vi "Increment Stage.vi"(11 "Circle the Wagons in":refnum<class "Circle the Wagons.lvclass">) -> (3 "Circle the Wagons out":refnum<class "Circle the Wagons.lvclass">)   [LabVIEW 2015, in "Circle the Wagons.lvclass"]
uses:
  Circle the Wagons.lvclass
  Circle the Wagons.lvclass/Circle the Wagons.ctl
  SubVIs/Read-Only Globals.vi
  Square/Square.lvclass
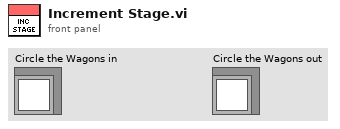
[diagram p1: front panel]
types:
  T1 = typedef "Circle the Wagons.lvclass/DVR Cluster.ctl" = cluster{"Stage":i32}
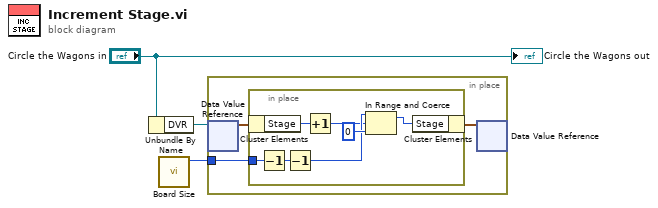
[diagram p0: block diagram]
diagram:
  n1 = Unbundle By Name("Circle the Wagons in") -> ("DVR"=w2:refnum<data-value>)
  n2 = call "Board Size.vi"() -> ("Board Size"=w1:i32)  [unwired: 11 in]
  n3 = in-place {
    in-place-border: w1 -> [w4]
    n4 = in-place-dvr #1(w2) -> (w6:T1)  [unwired: 1 out]
    n5 = in-place {
      in-place-border: w4 -> [w10]
      n6 = in-place-cluster #2(w6) -> ("Stage"=w13:i32)
      n7 = Decrement(x=w10) -> (x-1=w9:i32)
      n8 = Decrement(x=w9) -> (x-1=w8:i32)
      n9 = Increment(x=w13) -> (x+1=w7:i32)
      n10 = In Range and Coerce(upper limit=w8, x=w7, lower limit=0) -> (coerced(x)=w11:i32)  [unwired: 1 out]
      n11 = in-place-cluster #2("Stage"=w11) -> (w5:T1)
    }
    n12 = in-place-dvr #1(w5) -> ()  [unwired: 2 out]
  }
  "Circle the Wagons out" <- "Circle the Wagons in"
